vi "Workspace.vi"() -> ()   [LabVIEW 2015]
uses:
  <vilib>/express/express analysis/Spectral/Block/exnSpectralBlock spectral measurements peak poly.vi
  <vilib>/express/express analysis/Spectral/Block/exnSpectralBlock spectral measurements peak DDT.vi
  <vilib>/imath/engines/lvmath2/RunTimeEngine/Managers/WorkSpace/UID Generator.vi
  <vilib>/imath/engines/lvmath2/RunTimeEngine/RunTimeType/NIMS_RunTimeType_From StrictType (excl LVString).vi
  <instcachedir>/0/NIMS_RunTimeType_From StrictType (excl LVString)_EB1C38A9BC5048DA9ABDA8F781E54D21.lvgen/NIMS_RunTimeType_From StrictType (excl LVString)_EB1C38A9BC5048DA9ABDA8F781E54D21_000.vi
  <vilib>/imath/engines/lvmath2/RunTimeEngine/RunTimeType/NIMS_RunTimeType_Set Source Original Bool.vi
  <vilib>/imath/engines/lvmath2/RunTimeEngine/LocalVariableDefStatement/MC_LocalVariableDefStatement_Display.vi
  <vilib>/imath/engines/lvmath2/RunTimeEngine/Managers/SymbolTable/Clear UID.vi
  <vilib>/imath/engines/lvmath2/RunTimeEngine/NodeEndStatement/NIMS_NodeEndStatement_Output.vi
  <instcachedir>/0/NIMS_NodeEndStatement_Output_53EC0D466D134D7ABD903AC30B43404B.lvgen/NIMS_NodeEndStatement_Output_53EC0D466D134D7ABD903AC30B43404B_012.vi
  <vilib>/imath/engines/lvmath2/RunTimeEngine/ErrorHandling/NIMS_Finalize Error.vi
  <vilib>/express/express analysis/Spectral/XNode/ExpressSpectralMeasurementsBlockNode.xnode
  <vilib>/imath/engines/lvmath2/RunTimeEngine/Managers/SymbolTable/NIMS_WorkSpace.lvlib
panel:
  out "Spectral Measurements 3":dynamicdata(graph)
  in  "Input Control 3":cluster{"# of samples":i32, "Rate":dbl}
  out "Aquired Signal 3":dynamicdata(graph)
  out "Tone Measurements 3":cluster{"Amplitude":dbl, "Frequency":dbl}
  out "Boolean 20":bool
  out "Waveform Graph 3":dynamicdata(graph)
  out "Boolean 19":bool
  out "Boolean 18":bool
  out "Boolean 17":bool
  in  "Boolean 16":bool
  in  "Boolean 15":bool
  out "Boolean 14":bool
  out "Boolean 13":bool
  in  "Boolean 12":bool
  in  "Boolean 11":bool
  out "Spectral Measurements 2":dynamicdata(graph)
  in  "Input Control 2":cluster{"# of samples":i32, "Rate":dbl}
  out "Aquired Signal 2":dynamicdata(graph)
  in  "stop 2":bool
  out "Tone Measurements 2":cluster{"Amplitude":dbl, "Frequency":dbl}
  out "Boolean 2":bool
  out "Waveform Graph 2":dynamicdata(graph)
  out "Spectral Measurements":dynamicdata(graph)
  in  "Input Control":cluster{"# of samples":i32, "Rate":dbl}
  out "Aquired Signal":dynamicdata(graph)
  in  "stop":bool
  out "Tone Measurements":cluster{"Amplitude":dbl, "Frequency":dbl}
  out "Boolean":bool
  out "Waveform Graph":dynamicdata(graph)
  out "Boolean 7":bool
  out "Boolean 8":bool
  in  "Boolean 9":bool
  in  "Boolean 10":bool
  out "Boolean 3":bool
  out "Boolean 4":bool
  in  "Boolean 6":bool
  in  "Boolean 5":bool
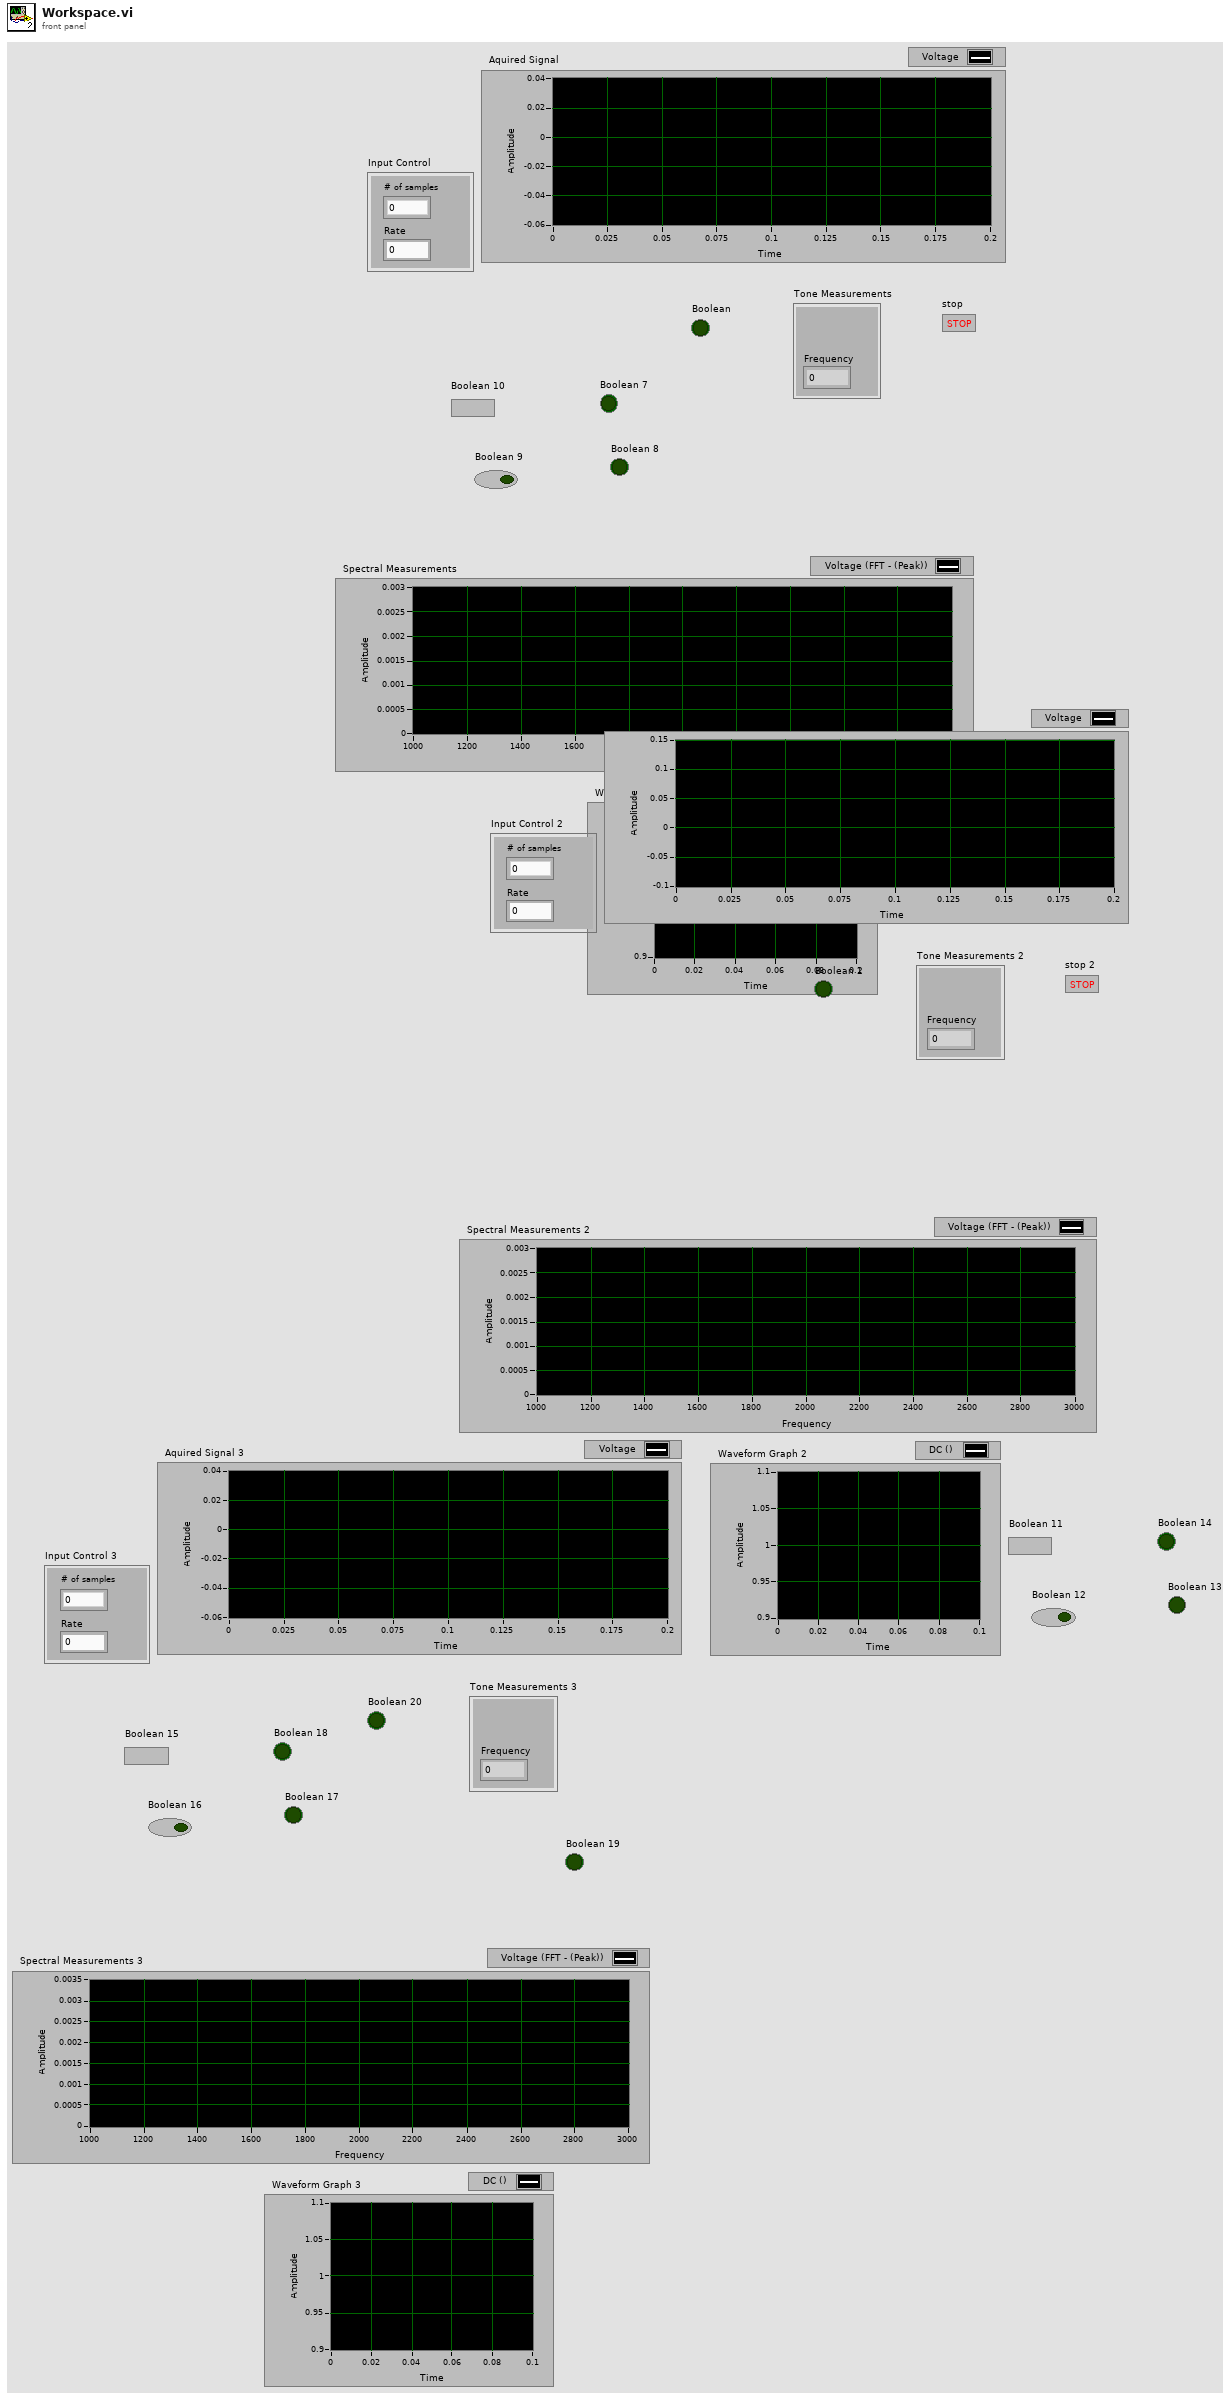
[diagram p1: front panel]
types:
  T1 = cluster{"averaging mode":u16, "weighting mode":u16, "number of averages":u32}
  T2 = cluster{"dB On (F)":bool, "unwrap phase (F)":bool, "convert to degree (F)":bool}
  T3 = cluster{"Amplitude":dynamicdata, "Frequency":dynamicdata}
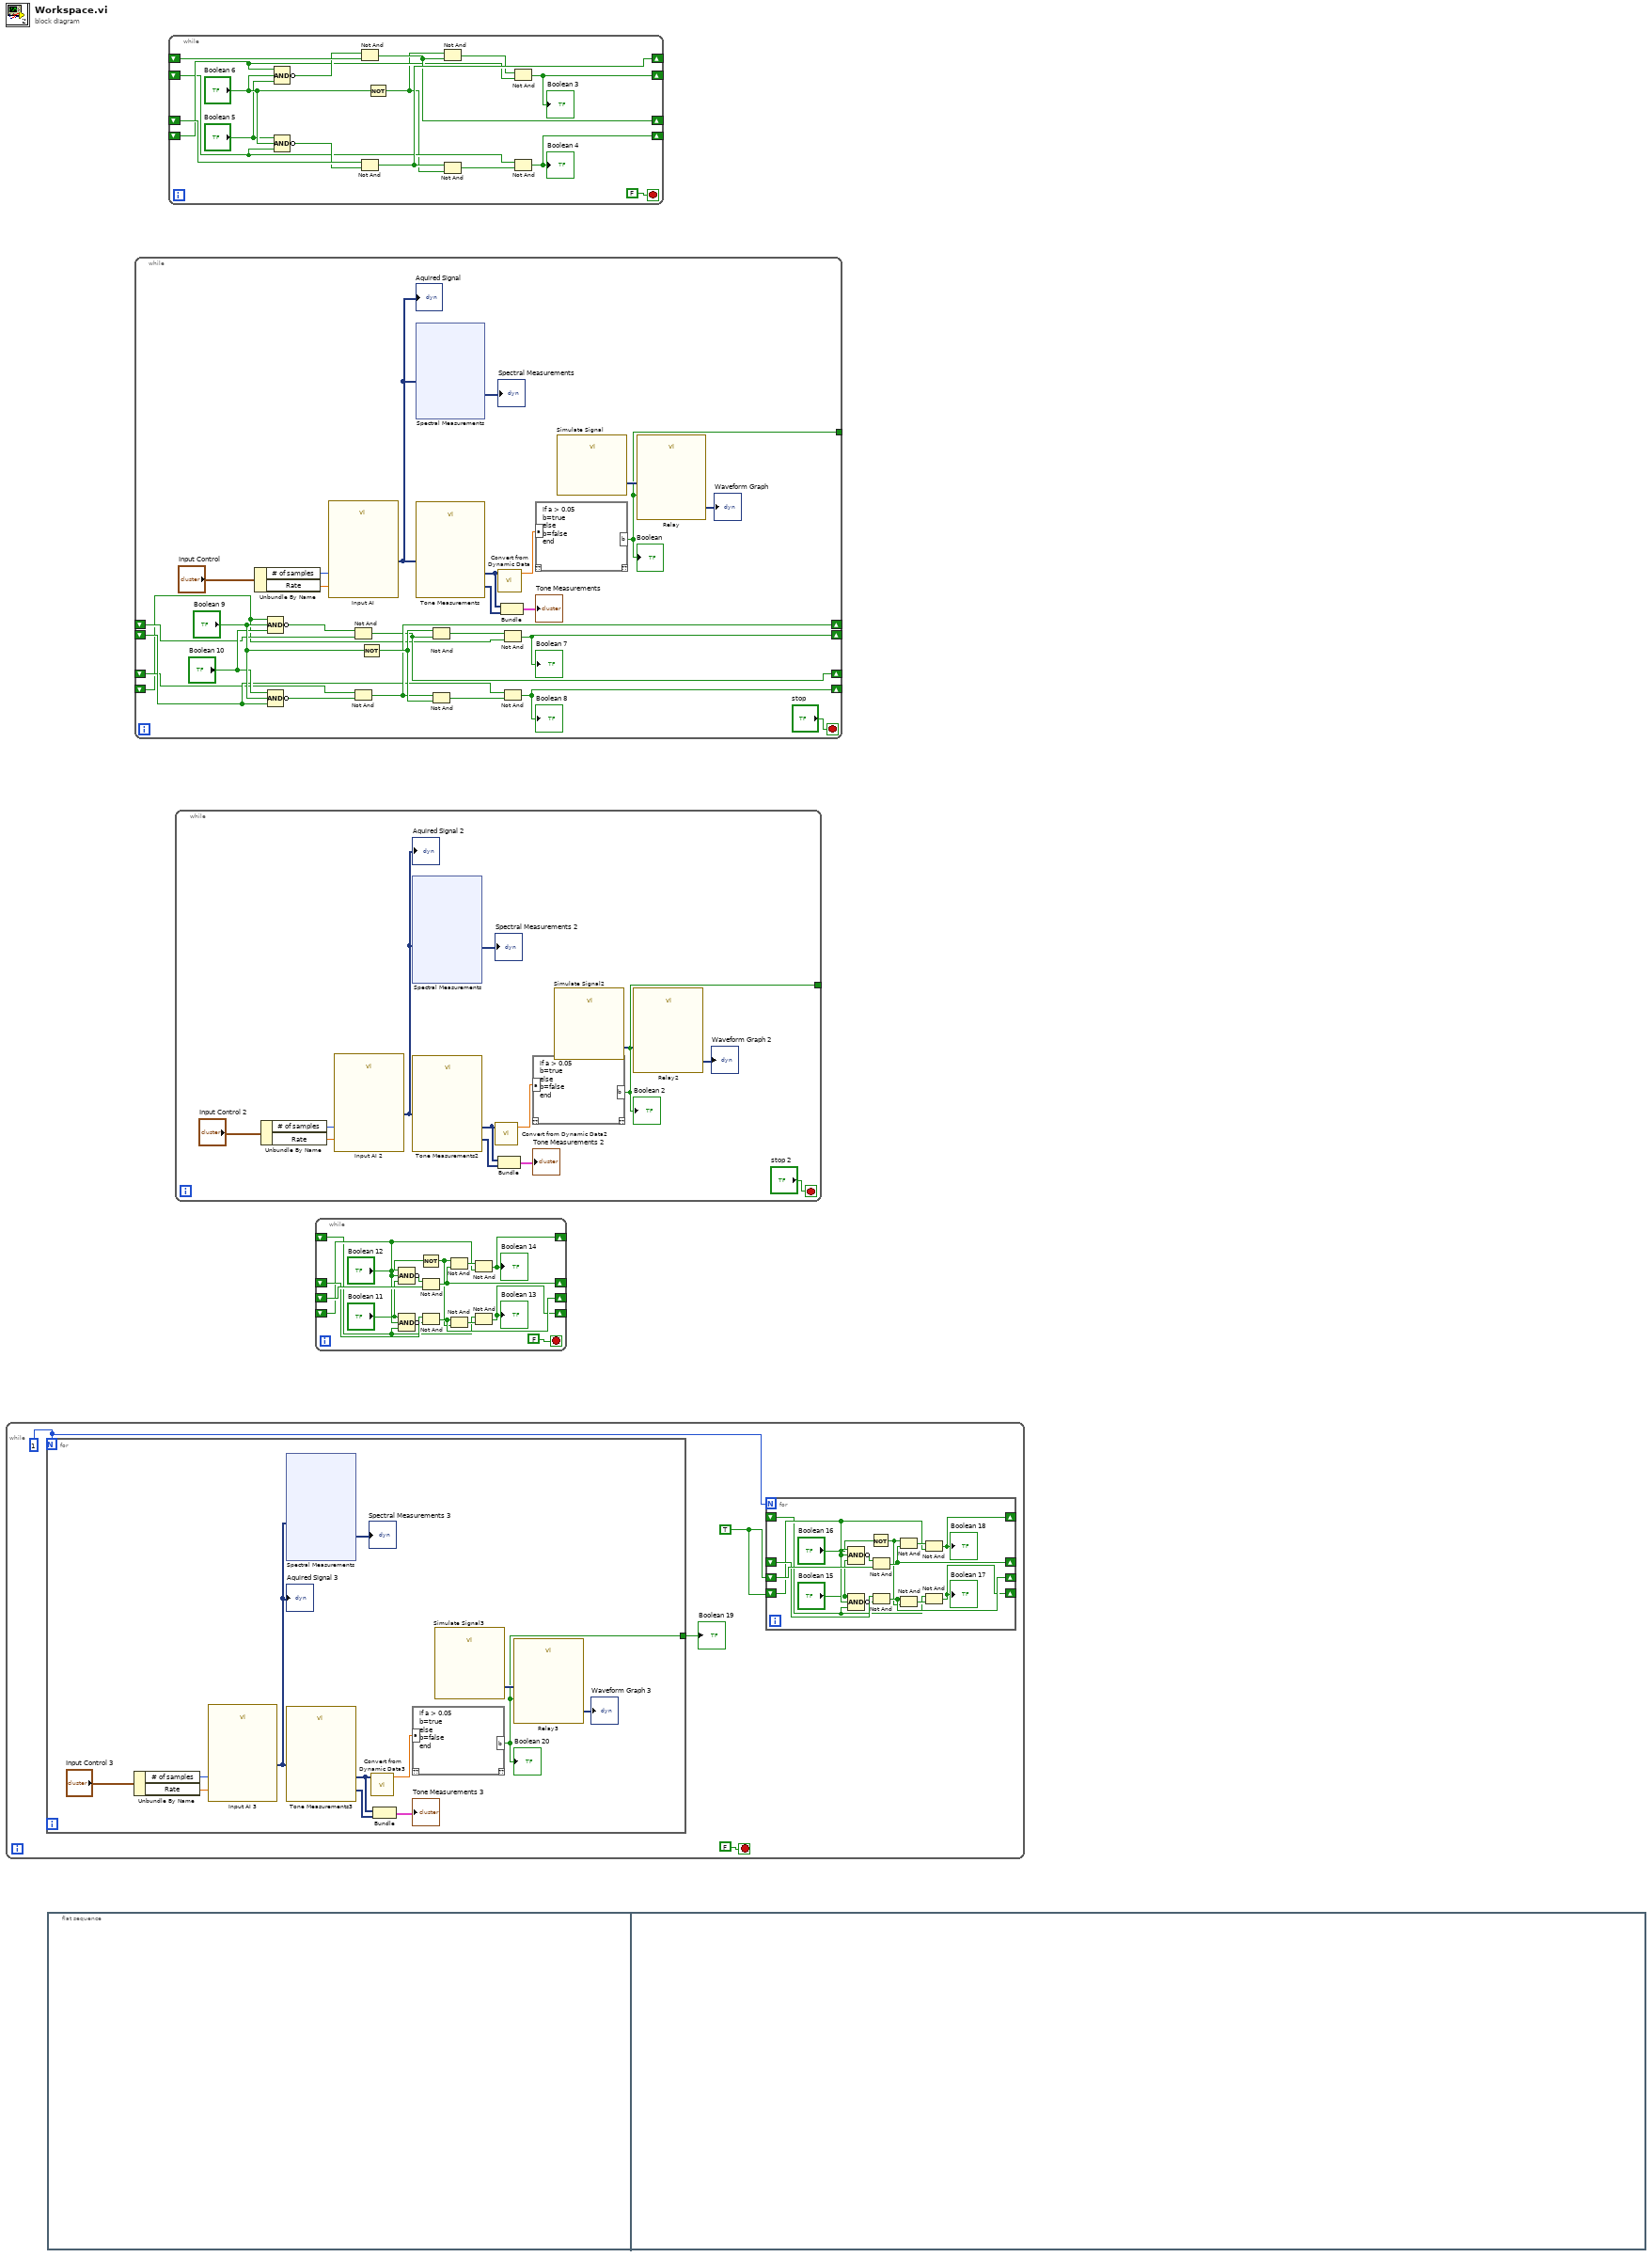
[diagram p0: block diagram]
diagram:
  n1 = while {
    stop <- FALSE stop-if-true
    w2 = TRUE
    w1 = 1
    n2 = for {
      N: w1 -> [_]
      tunnel: [w20] -> w3
      n3 = Unbundle By Name("Input Control 3") -> ("# of samples"=w22:i32, "Rate"=w23:dbl)
      n4 = call "Input AI 3"("rate"=w23, "number of samples"=w22) -> ("data"=w25:dynamicdata)  [unwired: 14 in, 3 out]
      "Aquired Signal 3" <- w25
      n5 = xnode "Spectral Measurements"("Signals"=w25) -> ("FFT - (Peak)"=→"Spectral Measurements 3":dynamicdata)  [unwired: 1 in, 2 out]
      n6 = call "Tone Measurements3"("Signals"=w25) -> ("Frequency"=w28:dynamicdata, "Amplitude"=w27:dynamicdata)  [unwired: 8 in, 1 out]
      n7 = call "Convert from Dynamic Data3"("Dynamic Data Type"=w27) -> ("Scalar"=w29:dbl)  [unwired: 3 in]
      n8 = Bundle("Amplitude"=w27, "Frequency"=w28) -> (→"Tone Measurements 3":T3)  [unwired: 1 in]
      n9 = mathscript code="if a > 0.05\nb=true\nelse\nb=false\nend"("a"=w29) -> ("b"=w20:bool)  [unwired: 1 in, 1 out]
      "Boolean 20" <- w20
      n10 = call "Simulate Signal3"() -> ("DC"=w30:dynamicdata)  [unwired: 14 in, 1 out]
      n11 = call "Relay3"("Enable"=w20, "Signals"=w30) -> ("Result"=→"Waveform Graph 3":dynamicdata)  [unwired: 8 in, 1 out]
    }
    "Boolean 19" <- w3
    n12 = for {
      N: w1 -> [_]
      shift-right: [w7] -> _
      shift-left: w2 -> [w11]
      shift-right: [w16] -> _
      shift-left: _ -> [w18]
      shift-right: [w8] -> _
      shift-left: _ -> [w10]
      shift-right: [w17] -> _
      shift-left: w2 -> [w19]
      n13 = Compound Arithmetic op=AND(w11, "Boolean 16", "Boolean 15") -> (invert w14:bool)
      n14 = Compound Arithmetic op=AND("Boolean 15", "Boolean 16", w10) -> (invert w15:bool)
      n15 = Not(x="Boolean 16") -> (.not. x?=w9:bool)
      n16 = Not And(1:w19, 2:w14) -> (0:w16:bool)
      n17 = Not And(1:w15, 2:w18) -> (0:w17:bool)
      n18 = Not And(1:w16, 2:w9) -> (0:w13:bool)
      n19 = Not And(1:w9, 2:w17) -> (0:w12:bool)
      n20 = Not And(1:w11, 2:w13) -> (0:w8:bool)
      "Boolean 18" <- w8
      n21 = Not And(1:w12, 2:w10) -> (0:w7:bool)
      "Boolean 17" <- w7
    }
  }
  n22 = flat-sequence {
    frame #0 {
    }
    frame #1 {
    }
  }
  n23 = while {
    tunnel: [w123] -> _
    shift-right: [w115] -> _
    shift-left: _ -> [w111]
    shift-right: [w114] -> _
    shift-left: _ -> [w110]
    shift-right: [w113] -> _
    shift-left: _ -> [w109]
    shift-right: [w112] -> _
    shift-left: _ -> [w108]
    stop <- "stop" stop-if-true
    n24 = Unbundle By Name("Input Control") -> ("# of samples"=w134:i32, "Rate"=w133:dbl)
    n25 = Compound Arithmetic op=AND(w108, "Boolean 9", "Boolean 10") -> (invert w121:bool)
    n26 = Compound Arithmetic op=AND("Boolean 10", "Boolean 9", w110) -> (invert w122:bool)
    n27 = call "Input AI"("rate"=w133, "number of samples"=w134) -> ("data"=w131:dynamicdata)  [unwired: 14 in, 3 out]
    "Aquired Signal" <- w131
    n28 = Not And(1:w111, 2:w121) -> (0:w113:bool)
    n29 = Not And(1:w122, 2:w109) -> (0:w115:bool)
    n30 = Not(x="Boolean 9") -> (.not. x?=w118:bool)
    n31 = xnode "Spectral Measurements"("Signals"=w131) -> ("FFT - (Peak)"=→"Spectral Measurements":dynamicdata)  [unwired: 1 in, 2 out]
    n32 = call "Tone Measurements"("Signals"=w131) -> ("Frequency"=w127:dynamicdata, "Amplitude"=w128:dynamicdata)  [unwired: 8 in, 1 out]
    n33 = Not And(1:w113, 2:w118) -> (0:w120:bool)
    n34 = Not And(1:w118, 2:w115) -> (0:w119:bool)
    n35 = call "Convert from Dynamic Data"("Dynamic Data Type"=w128) -> ("Scalar"=w126:dbl)  [unwired: 3 in]
    n36 = Bundle("Amplitude"=w128, "Frequency"=w127) -> (→"Tone Measurements":T3)  [unwired: 1 in]
    n37 = Not And(1:w108, 2:w120) -> (0:w114:bool)
    "Boolean 7" <- w114
    n38 = Not And(1:w119, 2:w110) -> (0:w112:bool)
    "Boolean 8" <- w112
    n39 = mathscript code="if a > 0.05\nb=true\nelse\nb=false\nend"("a"=w126) -> ("b"=w123:bool)  [unwired: 1 in, 1 out]
    "Boolean" <- w123
    n40 = call "Simulate Signal"() -> ("DC"=w125:dynamicdata)  [unwired: 14 in, 1 out]
    n41 = call "Relay"("Enable"=w123, "Signals"=w125) -> ("Result"=→"Waveform Graph":dynamicdata)  [unwired: 8 in, 1 out]
  }
  n42 = while {
    shift-right: [w214] -> _
    shift-left: _ -> [w218]
    shift-right: [w223] -> _
    shift-left: _ -> [w225]
    shift-right: [w215] -> _
    shift-left: _ -> [w217]
    shift-right: [w224] -> _
    shift-left: _ -> [w226]
    stop <- FALSE stop-if-true
    n43 = Compound Arithmetic op=AND(w218, "Boolean 6", "Boolean 5") -> (invert w221:bool)
    n44 = Compound Arithmetic op=AND("Boolean 5", "Boolean 6", w217) -> (invert w222:bool)
    n45 = Not And(1:w226, 2:w221) -> (0:w223:bool)
    n46 = Not And(1:w222, 2:w225) -> (0:w224:bool)
    n47 = Not(x="Boolean 6") -> (.not. x?=w216:bool)
    n48 = Not And(1:w223, 2:w216) -> (0:w220:bool)
    n49 = Not And(1:w216, 2:w224) -> (0:w219:bool)
    n50 = Not And(1:w218, 2:w220) -> (0:w215:bool)
    "Boolean 3" <- w215
    n51 = Not And(1:w219, 2:w217) -> (0:w214:bool)
    "Boolean 4" <- w214
  }
  n52 = while {
    tunnel: [w228] -> _
    stop <- "stop 2" stop-if-true
    n53 = Unbundle By Name("Input Control 2") -> ("# of samples"=w239:i32, "Rate"=w238:dbl)
    n54 = call "Input AI 2"("rate"=w238, "number of samples"=w239) -> ("data"=w236:dynamicdata)  [unwired: 14 in, 3 out]
    "Aquired Signal 2" <- w236
    n55 = xnode "Spectral Measurements"("Signals"=w236) -> ("FFT - (Peak)"=→"Spectral Measurements 2":dynamicdata)  [unwired: 1 in, 2 out]
    n56 = call "Tone Measurements2"("Signals"=w236) -> ("Frequency"=w232:dynamicdata, "Amplitude"=w233:dynamicdata)  [unwired: 8 in, 1 out]
    n57 = call "Convert from Dynamic Data2"("Dynamic Data Type"=w233) -> ("Scalar"=w231:dbl)  [unwired: 3 in]
    n58 = Bundle("Amplitude"=w233, "Frequency"=w232) -> (→"Tone Measurements 2":T3)  [unwired: 1 in]
    n59 = mathscript code="if a > 0.05\nb=true\nelse\nb=false\nend"("a"=w231) -> ("b"=w228:bool)  [unwired: 1 in, 1 out]
    "Boolean 2" <- w228
    n60 = call "Simulate Signal2"() -> ("DC"=w230:dynamicdata)  [unwired: 14 in, 1 out]
    n61 = call "Relay2"("Enable"=w228, "Signals"=w230) -> ("Result"=→"Waveform Graph 2":dynamicdata)  [unwired: 8 in, 1 out]
  }
  n62 = while {
    shift-right: [w319] -> _
    shift-left: _ -> [w323]
    shift-right: [w328] -> _
    shift-left: _ -> [w330]
    shift-right: [w320] -> _
    shift-left: _ -> [w322]
    shift-right: [w329] -> _
    shift-left: _ -> [w331]
    stop <- FALSE stop-if-true
    n63 = Compound Arithmetic op=AND(w323, "Boolean 12", "Boolean 11") -> (invert w326:bool)
    n64 = Compound Arithmetic op=AND("Boolean 11", "Boolean 12", w322) -> (invert w327:bool)
    n65 = Not(x="Boolean 12") -> (.not. x?=w321:bool)
    n66 = Not And(1:w331, 2:w326) -> (0:w328:bool)
    n67 = Not And(1:w327, 2:w330) -> (0:w329:bool)
    n68 = Not And(1:w328, 2:w321) -> (0:w325:bool)
    n69 = Not And(1:w321, 2:w329) -> (0:w324:bool)
    n70 = Not And(1:w323, 2:w325) -> (0:w320:bool)
    "Boolean 14" <- w320
    n71 = Not And(1:w324, 2:w322) -> (0:w319:bool)
    "Boolean 13" <- w319
  }
